vi "DefineRect.vi"(10 "cell size":i32, 11 "Cell in":refnum<class "Cell.lvclass">) -> (3 "Cell out":refnum<class "Cell.lvclass">)   [LabVIEW 2021, in "Cell.lvclass"]
uses:
  Cell.lvclass
  Cell.lvclass/Cell.ctl
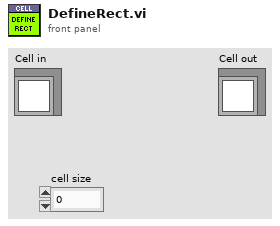
[diagram p1: front panel]
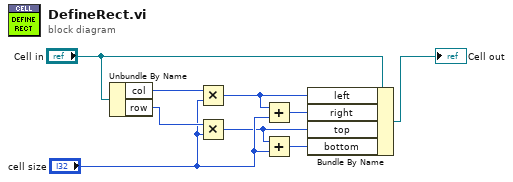
[diagram p0: block diagram]
diagram:
  n1 = Unbundle By Name("Cell in") -> ("col"=w8:i32, "row"=w7:i32)
  n2 = Multiply(x=w8, y="cell size") -> (x*y=w6:i32)
  n3 = Multiply(x=w7, y="cell size") -> (x*y=w1:i32)
  n4 = Add(x=w6, y="cell size") -> (x+y=w5:i32)
  n5 = Add(x=w1, y="cell size") -> (x+y=w4:i32)
  n6 = Bundle By Name(cluster="Cell in", "left"=w6, "right"=w5, "top"=w1, "bottom"=w4) -> (→"Cell out":refnum<class "Cell.lvclass">)
